vi "Secondary Joystick Control.vi"   [LabVIEW 2013]
types:
  T1 = typedef "WPI_JoystickButtonState.ctl" = cluster{"Button 1":bool, "Button 2":bool, "Button 3":bool, "Button 4":bool, "Button 5":bool, "Button 6":bool, "Button 7":bool, "Button 8":bool, "Button 9":bool, "Button 10":bool, "Button 11":bool, "Button 12":bool}
  T2 = cluster{"Axes":cluster{"X Axis":dbl, "Y Axis":dbl, "Throttle":dbl, "Unused":dbl, "Unused":dbl, "Unused":dbl}, "Buttons":T1}
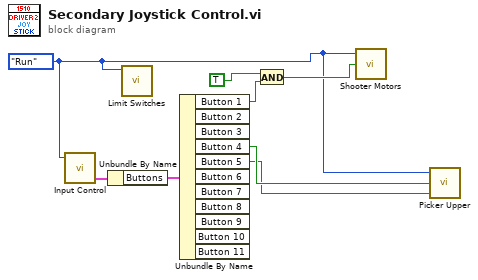
[diagram p0: block diagram]
diagram:
  w4 = enum16{"Open", "Run", "End"}."Run" ("State")
  n1 = call "Input Control.vi"("State"=w4) -> ("Secondary Joystick"=w8:T2)  [unwired: 2 in, 2 out]
  n2 = Unbundle By Name(w8) -> ("Buttons"=w7:T1)
  n3 = call "Limit Switches.vi"("State Control"=w4) -> ()  [unwired: 7 in, 4 out]
  n4 = Unbundle By Name(w7) -> ("Button 1"=w6:bool, "Button 4"=w3:bool, "Button 5"=w2:bool)  [unwired: 8 out]
  n5 = And(x=TRUE, y=w6) -> (x .and. y?=w5:bool)
  n6 = call "Shooter Motors.vi"("Fire"=w5, "State Control"=w4) -> ()  [unwired: 1 in]
  n7 = call "Picker Upper.vi"("Up"=w2, "Down"=w3, "State Control"=w4) -> ()
